vi "Set measured exp.vi"(8 "error in (no error)":errorcluster, 10 "Experiment":refnum<class "Experiment.lvclass">, 11 "Control-Client in":refnum<class "Control-Client.lvclass">) -> (0 "error out":errorcluster, 3 "Control-Client out":refnum<class "Control-Client.lvclass">)   [LabVIEW 2015, in "Control-Client.lvclass"]
uses:
  Control-Client.lvclass
  Experiments/Experiment.lvclass
  Control-Client.lvclass/Control-Client.ctl
  methods/Read Group #.vi
  Experiments/Experiments_group.lvclass
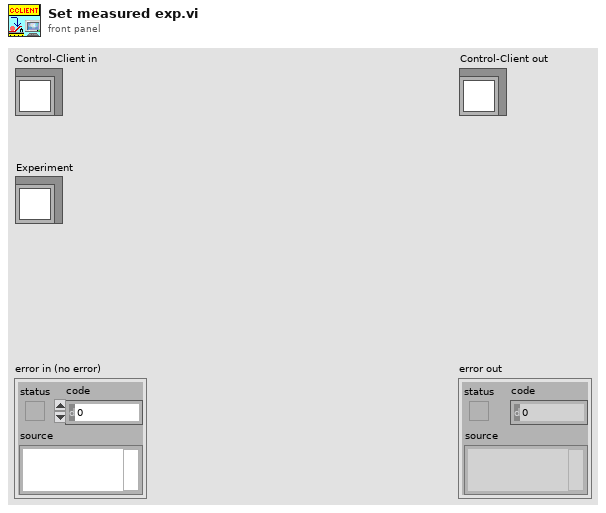
[diagram p1: front panel]
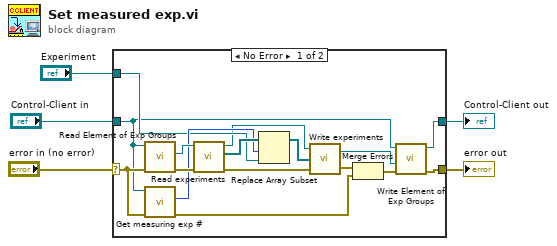
[diagram p0: block diagram]
diagram:
  n1 = case shown="No Error" "error in (no error)" {
    selector: "error in (no error)" -> [w21 w23]
    tunnel: [w12 w23] -> w4
    tunnel: [w11 w22] -> w2
    tunnel: "Control-Client in" -> [w14 w22]
    tunnel: "Experiment" -> [w15 _]
    frame No Error {
      n2 = call "Read Element of Exp Groups.vi"("error in (no error)"=w21, "Control-Client in"=w14) -> ("error out"=w19:errorcluster, "Experiments_group.lvclass"=w20:refnum<class "Experiments_group.lvclass">)  [unwired: 7 in, 1 out]
      n3 = call "Get measuring exp #.vi"("error in (no error)"=w21, "Control-Client in"=w14) -> ("error out"=w18:errorcluster, "Exp measure #"=w16:i32)  [unwired: 7 in, 1 out]
      n4 = call "Read experiments.vi"("error in (no error)"=w19, "Experiments_group.lvclass in"=w20) -> ("error out"=w8:errorcluster, "Experiments"=w17:refnum<class "Experiment.lvclass">[], "Experiments_group.lvclass out"=w10:refnum<class "Experiments_group.lvclass">)  [unwired: 6 in]
      n5 = Replace Array Subset(array=w17, new element=w15, index=w16) -> (w9:refnum<class "Experiment.lvclass">[])
      n6 = call-dynamic "Write experiments.vi"("error in (no error)"=w8, "Experiments"=w9, "Experiments_group.lvclass in"=w10) -> ("error out"=w7:errorcluster, "Experiments_group.lvclass out"=w6:refnum<class "Experiments_group.lvclass">)
      n7 = Merge Errors(w7, w18) -> (w13:errorcluster)
      n8 = call "Write Element of Exp Groups.vi"("error in (no error)"=w13, "Experiments_group.lvclass"=w6, "Control-Client in"=w14) -> ("error out"=w12:errorcluster, "Control-Client out"=w11:refnum<class "Control-Client.lvclass">)  [unwired: 7 in]
    }
    frame Error {
    }
  }
  "error out" <- w4
  "Control-Client out" <- w2
